vi "Pre-Actor.vi"(8 "error in (no error)":errorcluster, 11 "Fault Monitor in":refnum<class "Fault Monitor.lvclass">) -> (0 "error out":errorcluster, 3 "Fault Monitor out":refnum<class "Fault Monitor.lvclass">)   [LabVIEW 2023, in "Fault Monitor.lvlib" / "Fault Monitor.lvclass"]
doc: "<b>Pre-Actor </b>\nThis routine is called before registering for events, after control references have been mapped to the class private data. It is inteded to perform any additional actions before the actor front panel is displayed."
uses:
  Library/Fault Monitor.lvclass
  Library/Fault Monitor.lvclass/Fault Monitor.ctl
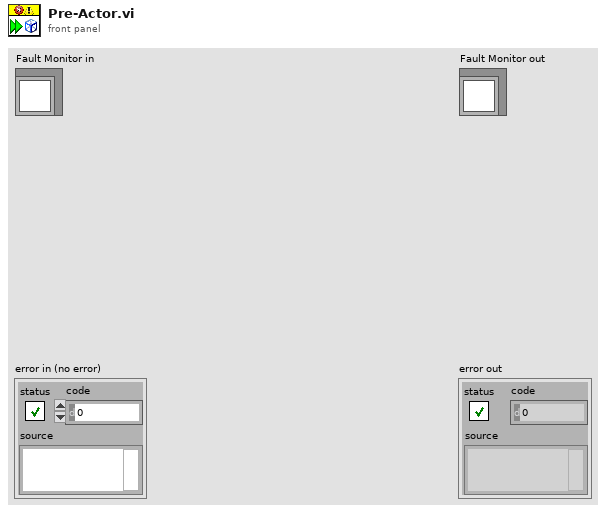
[diagram p1: front panel]
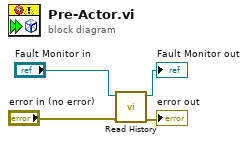
[diagram p0: block diagram]
diagram:
  n1 = call "Read History.vi"("error in (no error)"="error in (no error)", "Fault Monitor in"="Fault Monitor in") -> ("error out"=→"error out":errorcluster, "Fault Monitor out"=→"Fault Monitor out":refnum<class "Fault Monitor.lvclass">)  [unwired: 8 in]
